vi "ArthOps.vi"() -> ()   [LabVIEW 2026]
panel:
  out "x*y":dbl
  out "x-1":dbl
  out "x*2^n":dbl
  in  "x":dbl
  in  "y":dbl
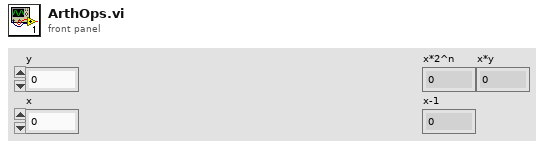
[diagram p1: front panel]
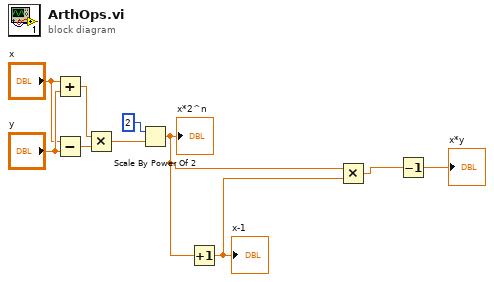
[diagram p0: block diagram]
diagram:
  n1 = Add(x="x", y="y") -> (x+y=w8:dbl)
  n2 = Subtract(x="x", y="y") -> (x-y=w7:dbl)
  n3 = Multiply(x=w8, y=w7) -> (x*y=w6:dbl)
  n4 = Scale By Power Of 2(n=i16 2, x=w6) -> (x*2^n=w4:dbl)
  "x*2^n" <- w4
  n5 = Increment(x=w4) -> (x+1=w3:dbl)
  "x-1" <- w3
  n6 = Multiply(x=w4, y=w3) -> (x*y=w2:dbl)
  n7 = Decrement(x=w2) -> (x-1=→"x*y":dbl)
